vi "VersionMutationFilenames.vi"(11 "New BlueSerializableVersion":u16) -> (1 "Mutate_v2_to_v3.vi":string, 2 "Mutate_v1_to_v2.vi":string, 3 "SerializableData_v2.ctl":string)   [LabVIEW 2019, in "BlueSerializationScripts.lvlib"]
uses:
  BlueSerializationScripts.lvlib
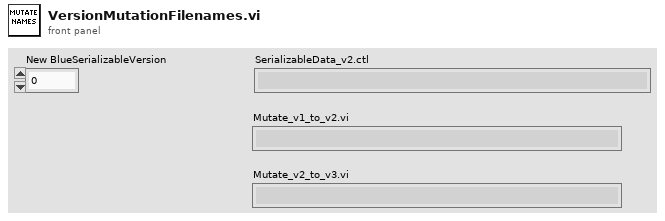
[diagram p1: front panel]
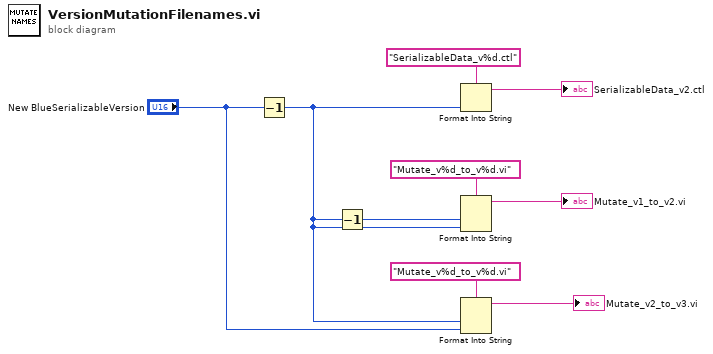
[diagram p0: block diagram]
diagram:
  n1 = Decrement(x="New BlueSerializableVersion") -> (x-1=w1:u16)
  n2 = Decrement(x=w1) -> (x-1=w2:u16)
  n3 = Format Into String(format string="SerializableData_v%d.ctl", w1) -> (resulting string=→"SerializableData_v2.ctl":string)  [unwired: 2 in, 1 out]
  n4 = Format Into String(format string="Mutate_v%d_to_v%d.vi", w2, w1) -> (resulting string=→"Mutate_v1_to_v2.vi":string)  [unwired: 2 in, 1 out]
  n5 = Format Into String(format string="Mutate_v%d_to_v%d.vi", w1, "New BlueSerializableVersion") -> (resulting string=→"Mutate_v2_to_v3.vi":string)  [unwired: 2 in, 1 out]
